vi "LVCAM Nest Destroyed.vi"(10 "Nest Actor":refnum<class "LVCAM.lvclass">, 11 "LVCAM Nest Destroyed in":refnum<class "LVCAM Nest Destroyed.lvclass">) -> (0 "error out":errorcluster, 3 "LVCAM Nest Destroyed out":refnum<class "LVCAM Nest Destroyed.lvclass">)   [LabVIEW 2021, in "LVCAM Nest Destroyed.lvlib" / "LVCAM Nest Destroyed.lvclass"]
uses:
  LVCAM Nest Destroyed.lvclass
  LVCAM/LVCAM/LVCAM.lvclass
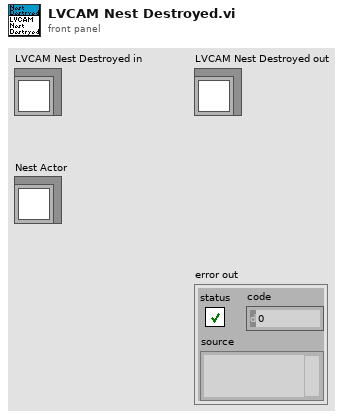
[diagram p1: front panel]
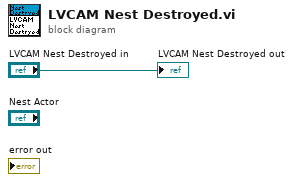
[diagram p0: block diagram]
diagram:
  "LVCAM Nest Destroyed out" <- "LVCAM Nest Destroyed in"
